vi "SCADA.vi"() -> ()   [LabVIEW 2014]
panel:
  in  "HAND AUTO":bool
  out "B4":bool
  out "B5":bool
  out "B1":bool
  out "B2":bool
  out "B3":bool
  out "PUMP 1 ON":bool
  out "PUMP 2 ON":bool
  out "INFLOW ON":bool
  out "FAULT":bool
  out "H PUMPS ON":bool
  out "A SYSTEM ON":bool
  in  "ACK":bool
  in  "E STOP":bool
  in  "H PUMPS OFF":bool
  in  "H PUMPS ON":bool
  in  "A SYSTEM OFF":bool
  in  "A SYSTEM ON":bool
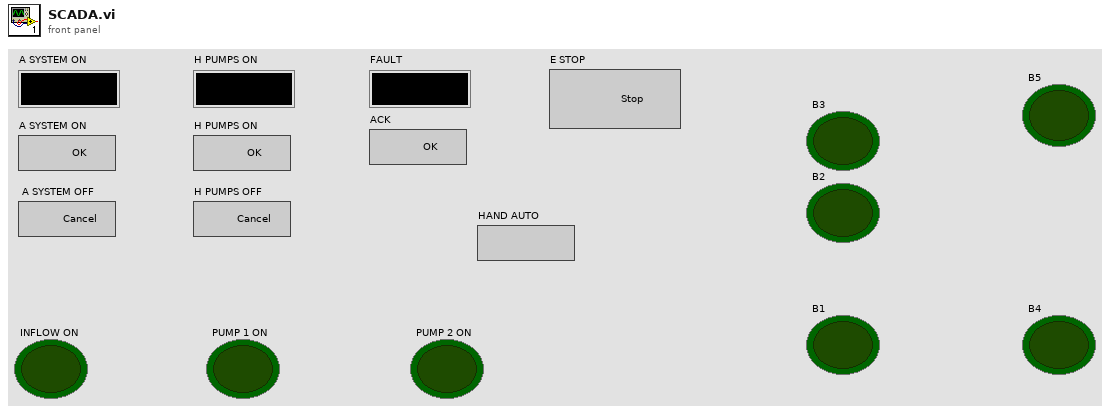
[diagram p1: front panel]
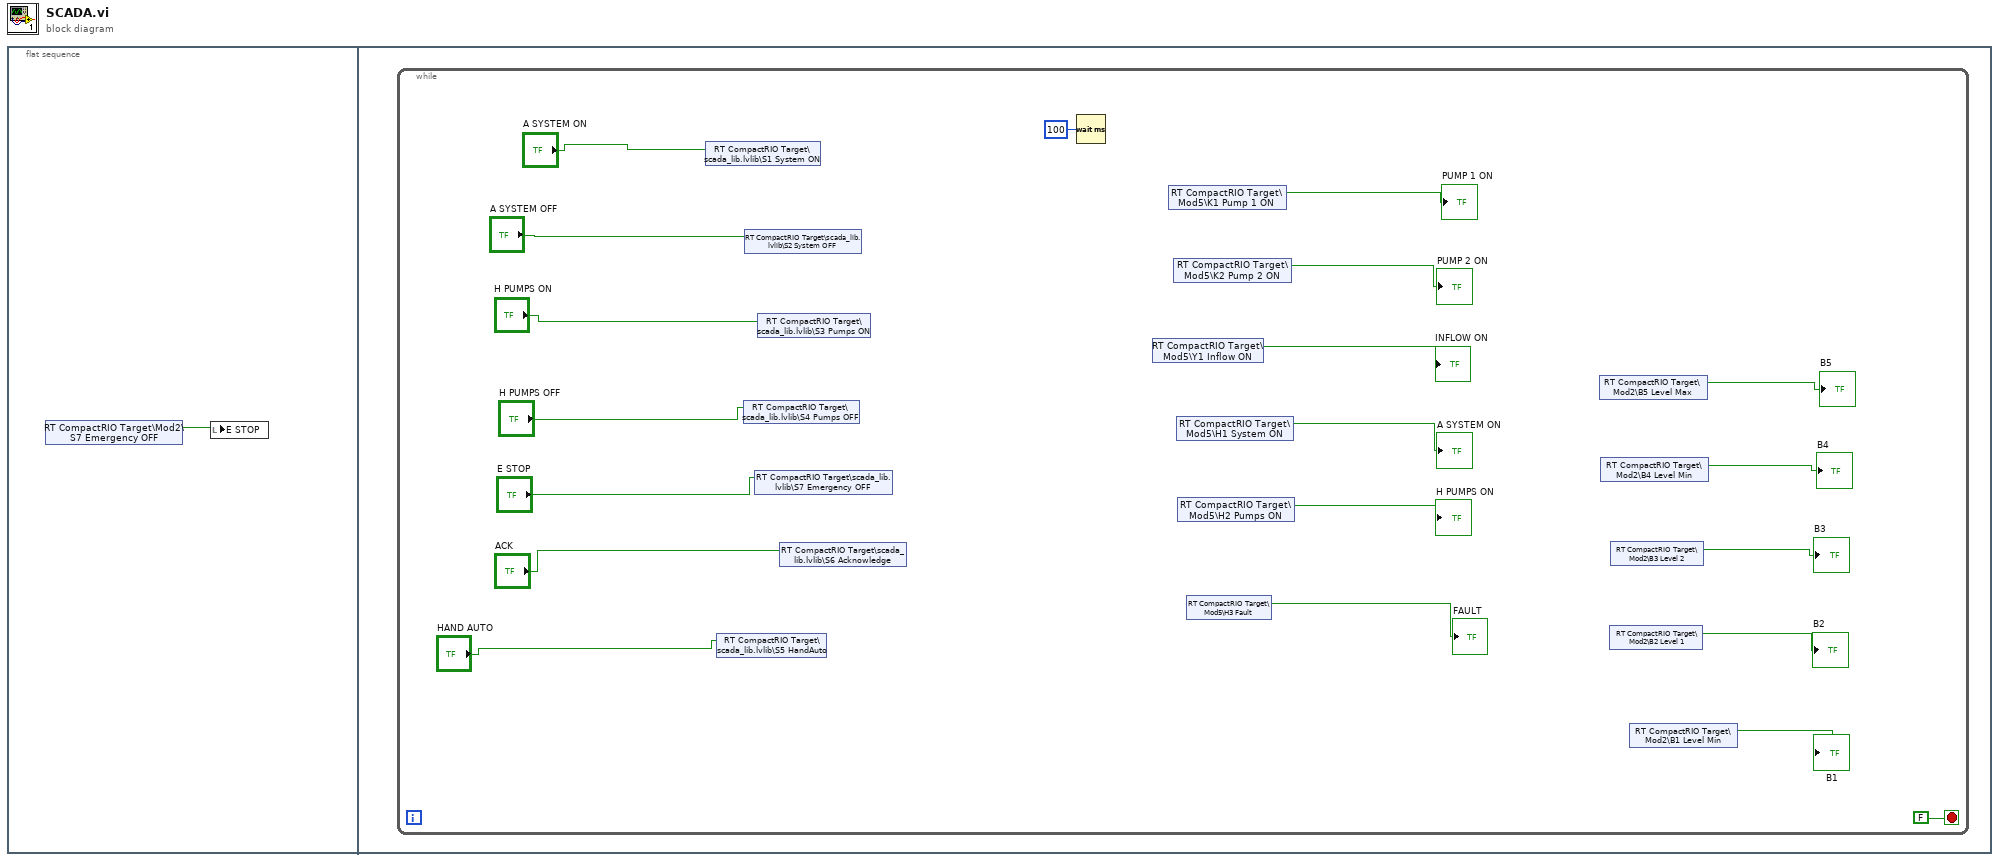
[diagram p0: block diagram]
diagram:
  n1 = flat-sequence {
    frame #0 {
      n2 = shared-variable "RT CompactRIO Target\\Mod2\\S7 Emergency OFF"() -> (w1:bool)  [unwired: 1 in, 1 out]
      n3 = local write "E STOP"(w1) -> ()
    }
    frame #1 {
      n4 = while {
        stop <- FALSE stop-if-true
        n5 = shared-variable "RT CompactRIO Target\\scada_lib.lvlib\\S1 System ON"("A SYSTEM ON") -> ()  [unwired: 1 in, 1 out]
        n6 = shared-variable "RT CompactRIO Target\\scada_lib.lvlib\\S5 HandAuto"("HAND AUTO") -> ()  [unwired: 1 in, 1 out]
        n7 = shared-variable "RT CompactRIO Target\\scada_lib.lvlib\\S4 Pumps OFF"("H PUMPS OFF") -> ()  [unwired: 1 in, 1 out]
        n8 = shared-variable "RT CompactRIO Target\\scada_lib.lvlib\\S2 System OFF"("A SYSTEM OFF") -> ()  [unwired: 1 in, 1 out]
        n9 = shared-variable "RT CompactRIO Target\\scada_lib.lvlib\\S7 Emergency OFF"("E STOP") -> ()  [unwired: 1 in, 1 out]
        n10 = shared-variable "RT CompactRIO Target\\scada_lib.lvlib\\S3 Pumps ON"("H PUMPS ON") -> ()  [unwired: 1 in, 1 out]
        n11 = shared-variable "RT CompactRIO Target\\scada_lib.lvlib\\S6 Acknowledge"("ACK") -> ()  [unwired: 1 in, 1 out]
        n12 = Wait (ms)(milliseconds to wait=u32 100) -> ()  [unwired: 1 out]
        n13 = shared-variable "RT CompactRIO Target\\Mod5\\Y1 Inflow ON"() -> (→"INFLOW ON":bool)  [unwired: 1 in, 1 out]
        n14 = shared-variable "RT CompactRIO Target\\Mod5\\K1 Pump 1 ON"() -> (→"PUMP 1 ON":bool)  [unwired: 1 in, 1 out]
        n15 = shared-variable "RT CompactRIO Target\\Mod5\\K2 Pump 2 ON"() -> (→"PUMP 2 ON":bool)  [unwired: 1 in, 1 out]
        n16 = shared-variable "RT CompactRIO Target\\Mod5\\H1 System ON"() -> (→"A SYSTEM ON":bool)  [unwired: 1 in, 1 out]
        n17 = shared-variable "RT CompactRIO Target\\Mod5\\H2 Pumps ON"() -> (→"H PUMPS ON":bool)  [unwired: 1 in, 1 out]
        n18 = shared-variable "RT CompactRIO Target\\Mod5\\H3 Fault"() -> (→"FAULT":bool)  [unwired: 1 in, 1 out]
        n19 = shared-variable "RT CompactRIO Target\\Mod2\\B5 Level Max"() -> (→"B5":bool)  [unwired: 1 in, 1 out]
        n20 = shared-variable "RT CompactRIO Target\\Mod2\\B4 Level Min"() -> (→"B4":bool)  [unwired: 1 in, 1 out]
        n21 = shared-variable "RT CompactRIO Target\\Mod2\\B2 Level 1"() -> (→"B2":bool)  [unwired: 1 in, 1 out]
        n22 = shared-variable "RT CompactRIO Target\\Mod2\\B3 Level 2"() -> (→"B3":bool)  [unwired: 1 in, 1 out]
        n23 = shared-variable "RT CompactRIO Target\\Mod2\\B1 Level Min"() -> (→"B1":bool)  [unwired: 1 in, 1 out]
      }
    }
  }
